vi "Write Numeric.vi"(8 "error in (no error)":errorcluster, 10 "Numeric":dbl, 11 "Math in":refnum<class "Math.lvclass">) -> (0 "error out":errorcluster, 3 "Math out":refnum<class "Math.lvclass">)   [LabVIEW 2016, in "Math.lvclass"]
uses:
  Math.lvclass
  Math.lvclass/Math.ctl
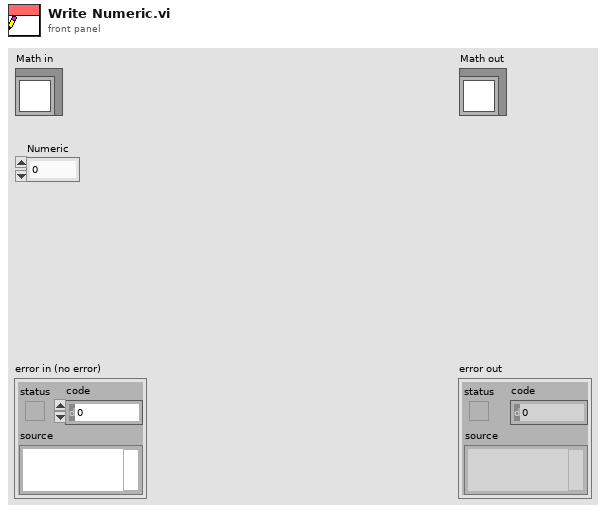
[diagram p1: front panel]
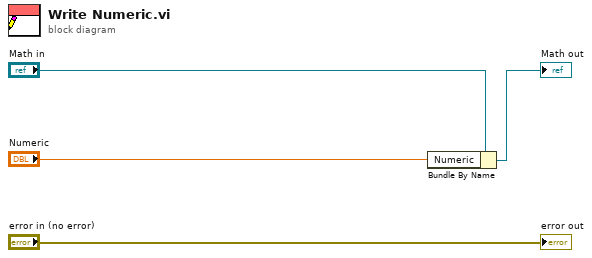
[diagram p0: block diagram]
diagram:
  n1 = Bundle By Name(cluster="Math in", "Numeric"="Numeric") -> (→"Math out":refnum<class "Math.lvclass">)
  "error out" <- "error in (no error)"
